vi "WBRT Read.vi"(8 "error in":errorcluster, 11 "WBRT State In":T2={"Encoders"={"Roll"=0.0, "Pitch"=0.0, "Yaw"=0.0, "Roll Trim"=0.0, "Pitch Trim"=0.0, "Yaw Trim"=0.0, "Roll Rate"=0.0, "Pitch Rate"=0.0, "Yaw Rate"=0.0}, "SPI Data"={"X-Gyro"=0.0, "Y-Gyro"=0.0, "Z-Gyro"=0.0, "X-Accel"=0.0, "Y-Accel"=0.0, "Z-Accel"=0.0}, "Camera"={"Numeric"=0.0}, "Filter Data"={"Filter Enabled?"=FALSE, "Filter Type"=enum."Equi-Ripple", "Pass Frequency"=1.0, "Stop Frequency (Equi-Ripple)"=0.45000000000000007, "Order"=0, "Ripple (dB)"=2.0}, "FPGA VI Reference"=refnum, "dt"=0.0, "Elapsed Time (msec)"=0, "Setpoints"={"Roll Setpoint (degrees)"=125.0, "Pitch Setpoint (degrees)"=125.0, "Yaw Setpoint (degrees)"=125.0}, "Commands"={"Left Command"=0.0, "Right Command"=0.0}, "Trajectory Data"=[], "Gains"={"Gain1"=0.0, "Gain2"=0.0, "Gain3"=0.0, "Gain4"=0.0, "Gain5"=0.0, "Gain6"=0.0, "Gain7"=0.0, "Gain8"=0.0, "Gain9"=0.0}, "Global Variables"={"Variable1"=[], "Variable2"=[], "Variable3"=[], "Variable4"=[]}, "Centroid"={"X Centroid"=0.0, "Y Centroid"=0.0}, "Error1"=0.0, "Error2"=0.0, "Error3"=0.0, "Error4"=0.0, "Recorded Data"=[], "Landing Factor"=0.0} {"Trajectory Data" format="%0.3f"; "Filter Data"."Stop Frequency (Equi-Ripple)" format="%0.3f"; "Filter Data"."Pass Frequency" format="%0.3f"}) -> (0 "error out":errorcluster, 2 "Chart Data":T1, 3 "WBRT State Out":T2={"Encoders"={"Roll"=0.0, "Pitch"=0.0, "Yaw"=0.0, "Roll Trim"=0.0, "Pitch Trim"=0.0, "Yaw Trim"=0.0, "Roll Rate"=0.0, "Pitch Rate"=0.0, "Yaw Rate"=0.0}, "SPI Data"={"X-Gyro"=0.0, "Y-Gyro"=0.0, "Z-Gyro"=0.0, "X-Accel"=0.0, "Y-Accel"=0.0, "Z-Accel"=0.0}, "Camera"={"Numeric"=0.0}, "Filter Data"={"Filter Enabled?"=FALSE, "Filter Type"=enum."Equi-Ripple", "Pass Frequency"=1.0, "Stop Frequency (Equi-Ripple)"=0.45000000000000007, "Order"=0, "Ripple (dB)"=2.0}, "FPGA VI Reference"=refnum, "dt"=0.0, "Elapsed Time (msec)"=0, "Setpoints"={"Roll Setpoint (degrees)"=125.0, "Pitch Setpoint (degrees)"=125.0, "Yaw Setpoint (degrees)"=125.0}, "Commands"={"Left Command"=0.0, "Right Command"=0.0}, "Trajectory Data"=[], "Gains"={"Gain1"=0.0, "Gain2"=0.0, "Gain3"=0.0, "Gain4"=0.0, "Gain5"=0.0, "Gain6"=0.0, "Gain7"=0.0, "Gain8"=0.0, "Gain9"=0.0}, "Global Variables"={"Variable1"=[], "Variable2"=[], "Variable3"=[], "Variable4"=[]}, "Centroid"={"X Centroid"=0.0, "Y Centroid"=0.0}, "Error1"=0.0, "Error2"=0.0, "Error3"=0.0, "Error4"=0.0, "Recorded Data"=[], "Landing Factor"=0.0} {"Trajectory Data" format="%0.3f"; "Filter Data"."Stop Frequency (Equi-Ripple)" format="%0.3f"; "Filter Data"."Pass Frequency" format="%0.3f"})   [LabVIEW 2012]
doc: "Reads and scales the encoder and IMU data.\n\nAuthor: Brandon Steele\n\nCopyright: Brigham Young University"
uses:
  Custom Controls/WBRT State.ctl
  Custom Controls/WBRT Encoders.ctl
  Custom Controls/WBRT SPI Data.ctl
  Custom Controls/WBRT Filter Data.ctl
  Custom Controls/WBRT Filter Type.ctl
  FPGA Samples/spi_single port_example/Host API/Controls/FPGA SPI_FPGA Ref.ctl
  Custom Controls/WBRT Setpoints.ctl
  Custom Controls/WBRT Commands.ctl
  Custom Controls/WBRT Gains.ctl
  Custom Controls/WBRT Global Variables.ctl
  <vilib>/Utility/error.llb/Error Cluster From Error Code.vi
  <vilib>/rvi/errors/niLvFpgaAdjustHostInterfaceError.vi
  <vilib>/rvi/interface/nirviReadWriteControl/nirviReadWriteControl.xnode
  FPGA Bitfiles/Whirlybird_FPGATarget_WhirlybirdFPGAMa_DBA2D843.lvbitx
  Whirlybird FPGA Main.vi
  NiFpgaLv.dll
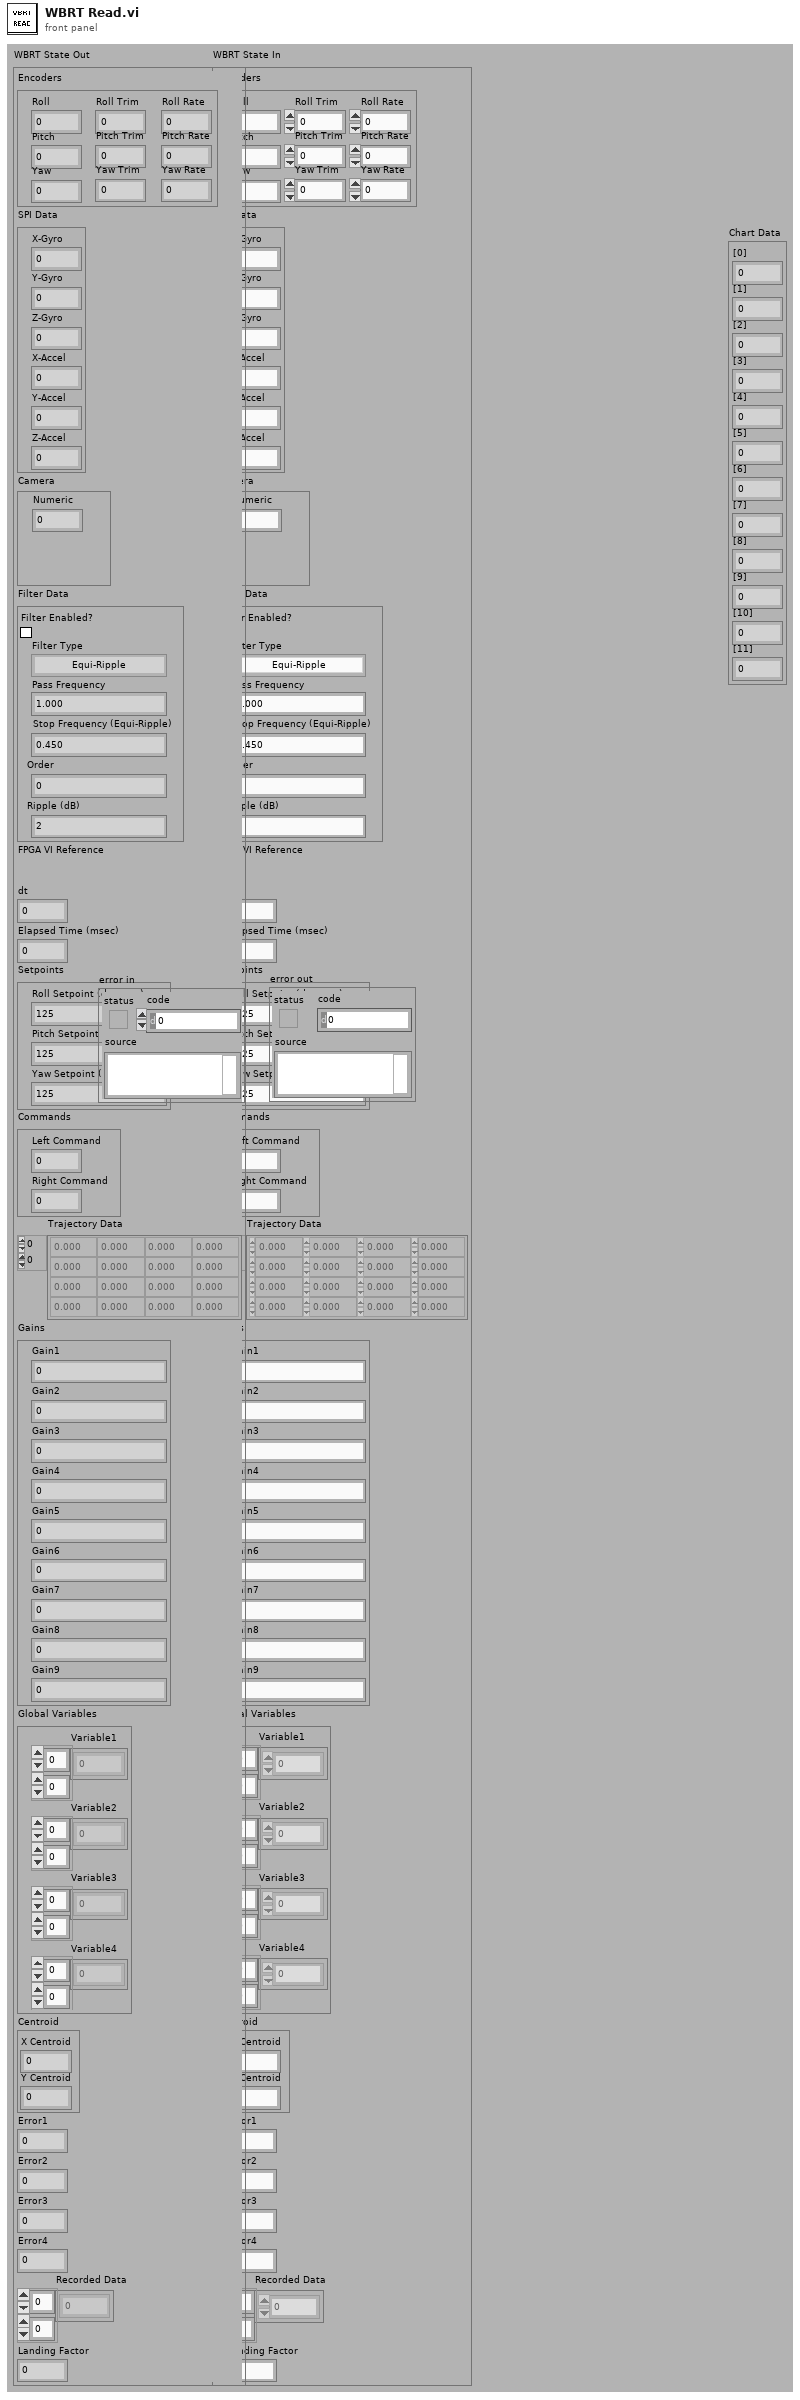
[diagram p1: front panel]
types:
  T1 = cluster{"[0]":dbl, "[1]":dbl, "[2]":dbl, "[3]":dbl, "[4]":dbl, "[5]":dbl, "[6]":dbl, "[7]":dbl, "[8]":dbl, "[9]":dbl, "[10]":dbl, "[11]":dbl}
  T2 = typedef "WBRT State.ctl" = cluster{"Encoders":T3, "SPI Data":T4, "Camera":cluster{"Numeric":dbl}, "Filter Data":T5, "FPGA VI Reference":T7, "dt":dbl, "Elapsed Time (msec)":u32, "Setpoints":T8, "Commands":T9, "Trajectory Data":dbl[][], "Gains":T10, "Global Variables":T11, "Centroid":cluster{"X Centroid":sgl, "Y Centroid":sgl}, "Error1":dbl, "Error2":dbl, "Error3":dbl, "Error4":dbl, "Recorded Data":dbl[][], "Landing Factor":dbl}
  T3 = typedef "WBRT Encoders.ctl" = cluster{"Roll":dbl, "Pitch":dbl, "Yaw":dbl, "Roll Trim":dbl, "Pitch Trim":dbl, "Yaw Trim":dbl, "Roll Rate":dbl, "Pitch Rate":dbl, "Yaw Rate":dbl}
  T4 = typedef "WBRT SPI Data.ctl" = cluster{"X-Gyro":dbl, "Y-Gyro":dbl, "Z-Gyro":dbl, "X-Accel":dbl, "Y-Accel":dbl, "Z-Accel":dbl}
  T5 = typedef "WBRT Filter Data.ctl" = cluster{"Filter Enabled?":bool, "Filter Type":T6, "Pass Frequency":dbl, "Stop Frequency (Equi-Ripple)":dbl, "Order":i32, "Ripple (dB)":dbl}
  T6 = typedef "WBRT Filter Type.ctl" = enum16{"Equi-Ripple", "Butterworth", "Chebyshev"}
  T7 = typedef "FPGA SPI_FPGA Ref.ctl" = refnum<k20>
  T8 = typedef "WBRT Setpoints.ctl" = cluster{"Roll Setpoint (degrees)":dbl, "Pitch Setpoint (degrees)":dbl, "Yaw Setpoint (degrees)":dbl}
  T9 = typedef "WBRT Commands.ctl" = cluster{"Left Command":dbl, "Right Command":dbl}
  T10 = typedef "WBRT Gains.ctl" = cluster{"Gain1":dbl, "Gain2":dbl, "Gain3":dbl, "Gain4":dbl, "Gain5":dbl, "Gain6":dbl, "Gain7":dbl, "Gain8":dbl, "Gain9":dbl}
  T11 = typedef "WBRT Global Variables.ctl" = cluster{"Variable1":dbl[][], "Variable2":dbl[][], "Variable3":dbl[][], "Variable4":dbl[][]}
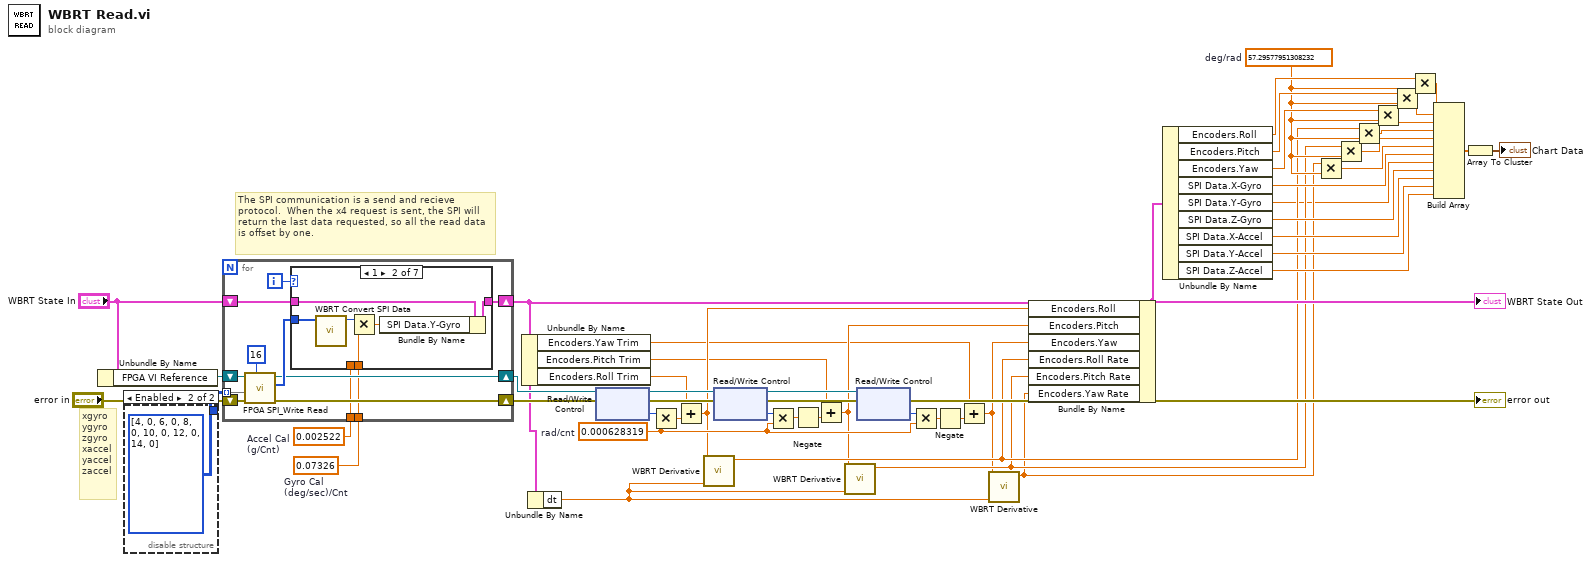
[diagram p0: block diagram]
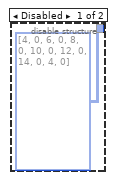
[diagram p2: hidden frame]
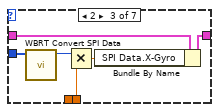
[diagram p4: hidden frame]
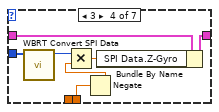
[diagram p5: hidden frame]
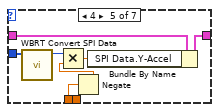
[diagram p6: hidden frame]
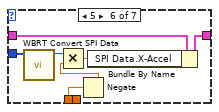
[diagram p7: hidden frame]
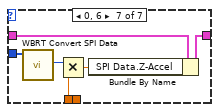
[diagram p8: hidden frame]
diagram:
  w9 = 0.002522  # Accel Cal (g/Cnt)
  w8 = 0.07326  # Gyro Cal (deg/sec)/Cnt
  w26 = 57.29577951308232  # deg/rad
  w36 = 0.000628319  # rad/cnt
  # "The SPI communication is a send and recieve protocol.  When the x4 request is sent, the SPI will return the last data requested, so all the read data is offset by one."
  # "xgyro\nygyro\nzgyro\nxaccel\nyaccel\nzaccel"
  n1 = Unbundle By Name("WBRT State In") -> ("FPGA VI Reference"=w52:T7)
  n2 = disable-structure shown="Enabled" {
    disable-tunnel: [u8[][] [[4, 0], [6, 0], [8, 0], [10, 0], [12, 0], [14, 0], [4, 0]] ("Write Data") u8[][] [[4, 0], [6, 0], [8, 0], [10, 0], [12, 0], [14, 0]] ("Write Data")] -> w51
    frame Disabled {
    }
    frame Enabled {
    }
  }
  n3 = for {
    tunnel: w51 -> [w65] mode=indexing
    shift-right: [w64] -> w48
    shift-left: "error in" -> [w63]
    shift-right: [w59] -> w7
    shift-left: "WBRT State In" -> [w60]
    shift-right: [w58] -> w47
    shift-left: w52 -> [w66]
    tunnel: w9 -> [w55]
    tunnel: w8 -> [w56]
    i -> [w62]
    n4 = call "FPGA SPI_Write Read.vi"("Total Bits"=u16 16, "error in"=w63, "Write Data"=w65, "FPGA VI Reference"=w66) -> ("error out"=w64:errorcluster, "Read Data"=w61:u8[], "FPGA VI Reference Out"=w58:T7)  [unwired: 5 in]
    n5 = case shown="1" w62 {
      tunnel: w61 -> [_ w71 w77 w84 w90 w97 w104]
      tunnel: w60 -> [w67 w73 w79 w86 w93 w100 w106]
      tunnel: [w67 w72 w78 w85 w92 w99 w105] -> w59
      tunnel: w56 -> [_ w69 w74 w81 _ _ _]
      tunnel: w55 -> [_ _ _ _ w88 w95 w101]
      frame Default {
        # "garbage data"
      }
      frame 1 {
        n6 = call "WBRT Convert SPI Data.vi"("Read Data"=w71) -> ("Value"=w70:i16)  [unwired: 10 in]
        n7 = Multiply(x=w70, y=w69) -> (x*y=w68:dbl)
        n8 = Bundle By Name(cluster=w73, "SPI Data.Y-Gyro"=w68) -> (w72:T2)
      }
      frame 2 {
        n9 = call "WBRT Convert SPI Data.vi"("Read Data"=w77) -> ("Value"=w76:i16)  [unwired: 10 in]
        n10 = Multiply(x=w76, y=w74) -> (x*y=w75:dbl)
        n11 = Bundle By Name(cluster=w79, "SPI Data.X-Gyro"=w75) -> (w78:T2)
      }
      frame 3 {
        n12 = call "WBRT Convert SPI Data.vi"("Read Data"=w84) -> ("Value"=w83:i16)  [unwired: 10 in]
        n13 = Negate(x=w81) -> (-x=w80:dbl)
        n14 = Multiply(x=w83, y=w80) -> (x*y=w82:dbl)
        n15 = Bundle By Name(cluster=w86, "SPI Data.Z-Gyro"=w82) -> (w85:T2)
      }
      frame 4 {
        n16 = call "WBRT Convert SPI Data.vi"("Read Data"=w90) -> ("Value"=w91:i16)  [unwired: 10 in]
        n17 = Negate(x=w88) -> (-x=w87:dbl)
        n18 = Multiply(x=w91, y=w87) -> (x*y=w89:dbl)
        n19 = Bundle By Name(cluster=w93, "SPI Data.Y-Accel"=w89) -> (w92:T2)
      }
      frame 5 {
        n20 = call "WBRT Convert SPI Data.vi"("Read Data"=w97) -> ("Value"=w98:i16)  [unwired: 10 in]
        n21 = Negate(x=w95) -> (-x=w94:dbl)
        n22 = Multiply(x=w98, y=w94) -> (x*y=w96:dbl)
        n23 = Bundle By Name(cluster=w100, "SPI Data.X-Accel"=w96) -> (w99:T2)
      }
      frame 0, 6 {
        n24 = call "WBRT Convert SPI Data.vi"("Read Data"=w104) -> ("Value"=w103:i16)  [unwired: 10 in]
        n25 = Multiply(x=w103, y=w101) -> (x*y=w102:dbl)
        n26 = Bundle By Name(cluster=w106, "SPI Data.Z-Accel"=w102) -> (w105:T2)
      }
    }
  }
  n27 = Unbundle By Name(w7) -> ("Encoders.Yaw Trim"=w1:dbl, "Encoders.Pitch Trim"=w3:dbl, "Encoders.Roll Trim"=w5:dbl)
  n28 = Unbundle By Name(w7) -> ("dt"=w27:dbl)
  n29 = xnode "Read/Write Control"("FPGA VI Reference In"=w47, "error in"=w48) -> ("FPGA VI Reference Out"=w45:T7, "error out"=w46:errorcluster, "Roll"=w39:i16)
  n30 = Multiply(x=w39, y=w36) -> (x*y=w29:dbl)
  n31 = Add(x=w5, y=w29) -> (x+y=w6:dbl)
  n32 = call "WBRT Derivative.vi"("dt"=w27, "Variable"=w6) -> ("Derivative"=w13:dbl)  [unwired: 9 in]
  n33 = xnode "Read/Write Control"("FPGA VI Reference In"=w45, "error in"=w46) -> ("FPGA VI Reference Out"=w43:T7, "error out"=w44:errorcluster, "Pitch"=w38:i16)
  n34 = Multiply(x=w38, y=w36) -> (x*y=w28:dbl)
  n35 = Negate(x=w28) -> (-x=w16:dbl)
  n36 = Add(x=w3, y=w16) -> (x+y=w4:dbl)
  n37 = call "WBRT Derivative.vi"("dt"=w27, "Variable"=w4) -> ("Derivative"=w12:dbl)  [unwired: 9 in]
  n38 = xnode "Read/Write Control"("FPGA VI Reference In"=w43, "error in"=w44) -> ("error out"=→"error out":errorcluster, "Yaw"=w37:i16)  [unwired: 1 out]
  n39 = Multiply(x=w37, y=w36) -> (x*y=w15:dbl)
  n40 = Negate(x=w15) -> (-x=w14:dbl)
  n41 = Add(x=w1, y=w14) -> (x+y=w2:dbl)
  n42 = call "WBRT Derivative.vi"("dt"=w27, "Variable"=w2) -> ("Derivative"=w11:dbl)  [unwired: 9 in]
  n43 = Bundle By Name(cluster=w7, "Encoders.Roll"=w6, "Encoders.Pitch"=w4, "Encoders.Yaw"=w2, "Encoders.Roll Rate"=w13, "Encoders.Pitch Rate"=w12, "Encoders.Yaw Rate"=w11) -> (w41:T2)
  "WBRT State Out" <- w41
  n44 = Unbundle By Name(w41) -> ("Encoders.Roll"=w35:dbl, "Encoders.Pitch"=w32:dbl, "Encoders.Yaw"=w30:dbl, "SPI Data.X-Gyro"=w22:dbl, "SPI Data.Y-Gyro"=w10:dbl, "SPI Data.Z-Gyro"=w21:dbl, "SPI Data.X-Accel"=w20:dbl, "SPI Data.Y-Accel"=w19:dbl, "SPI Data.Z-Accel"=w18:dbl)
  n45 = Multiply(x=w11, y=w26) -> (x*y=w23:dbl)
  n46 = Multiply(x=w12, y=w26) -> (x*y=w24:dbl)
  n47 = Multiply(x=w13, y=w26) -> (x*y=w25:dbl)
  n48 = Multiply(x=w30, y=w26) -> (x*y=w31:dbl)
  n49 = Multiply(x=w32, y=w26) -> (x*y=w33:dbl)
  n50 = Multiply(x=w35, y=w26) -> (x*y=w34:dbl)
  n51 = Build Array(w34, w33, w31, w25, w24, w23, w22, w10, w21, w20, w19, w18) -> (w40:dbl[])
  n52 = Array To Cluster(array=w40) -> (cluster=→"Chart Data":T1)
